vi "Add_Remove Point from Picture.vi"(6 "row index (0)":i32, 7 "2D Picture":refnum<vi>, 10 "draw options":T2={"Background Color"=16777215, "Grid Color"=13816530, "Angle Units"=enum."Degrees", "Draw Solid Background"=TRUE, "Draw Grid"=TRUE, "Grid Spacing"=0.25, "AutoScale"=FALSE, "Fit to Radius"=1.0, "data row options"=[]}, 11 "data in":T1) -> (0 "state changed?":bool, 1 "data changed?":bool, 3 "data out":T1)   [LabVIEW 2017, in "NI_Robotics_2D Rangefinder.xctl"]
uses:
  <vilib>/robotics/Controls/2D Rangefinder/NI_Robotics_2D Rangefinder.xctl
  <vilib>/robotics/Controls/2D Rangefinder/2D Rangefinder Picture/Draw Options.ctl
  <vilib>/robotics/Controls/Utilities/Angle Units.ctl
  <vilib>/robotics/Controls/2D Rangefinder/2D Rangefinder Picture/Data Row Options.ctl
  <vilib>/robotics/Controls/2D Rangefinder/2D Rangefinder Picture/Rangefinder Data.ctl
  <vilib>/robotics/Controls/2D Rangefinder/2D Rangefinder Picture/NI_Robotics_2D Rangefinder Picture.lvlib
  <vilib>/robotics/Controls/Utilities/NI_Robotics_Control Utilities.lvlib
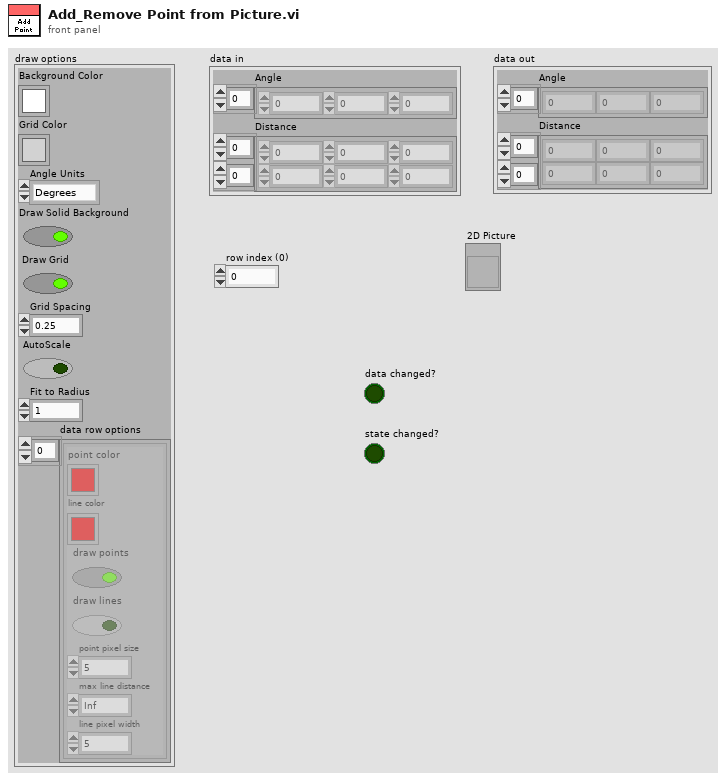
[diagram p1: front panel]
types:
  T1 = typedef "NI_Robotics_2D Rangefinder Picture.lvlib/Rangefinder Data.ctl" = cluster{"Angle":dbl[], "Distance":dbl[][]}
  T2 = typedef "NI_Robotics_2D Rangefinder Picture.lvlib/Draw Options.ctl" = cluster{"Background Color":u32, "Grid Color":u32, "Angle Units":T3, "Draw Solid Background":bool, "Draw Grid":bool, "Grid Spacing":dbl, "AutoScale":bool, "Fit to Radius":dbl, "data row options":T4[]}
  T3 = typedef "NI_Robotics_Control Utilities.lvlib/Angle Units.ctl" = enum16{"Radians", "Degrees"}
  T4 = typedef "NI_Robotics_2D Rangefinder Picture.lvlib/Data Row Options.ctl" = cluster{"point color":u32, "line color":u32, "draw points":bool, "draw lines":bool, "point pixel size":u16, "max line distance":dbl, "line pixel width":u16}
  T5 = typedef "LVBoundsTypeDef.ctl" = cluster{"Width":u32, "Height":u32}
  T6 = typedef "LVMouseTypeDef.ctl" = cluster{"Mouse Position":cluster{"X":i32, "Y":i32}, "Mouse Modifiers":cluster{"Button Down":bool, "Shift Mod":bool, "Menu Mod":bool, "Option Mod":bool}}
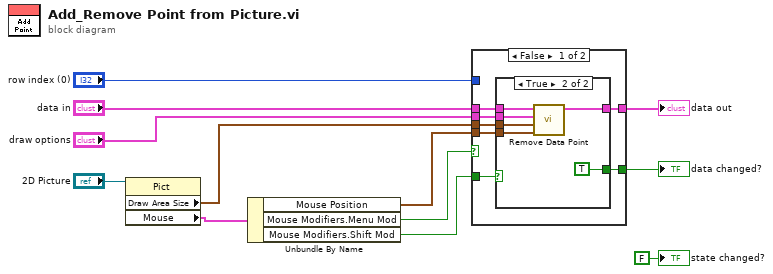
[diagram p0: block diagram]
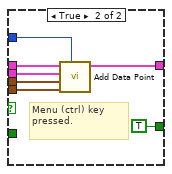
[diagram p3: hidden frame]
diagram:
  n1 = property class="Pict"(reference="2D Picture") -> ("Draw Area Size"=w10:T5, "Mouse"=w12:T6)  [unwired: 1 in, 2 out]
  n2 = Unbundle By Name(w12) -> ("Mouse Position"=w9:cluster{"X":i32, "Y":i32}, "Mouse Modifiers.Menu Mod"=w8:bool, "Mouse Modifiers.Shift Mod"=w7:bool)
  n3 = case shown="False" w8 {
    tunnel: "data in" -> [w18 w33]
    tunnel: [w17 w32] -> w2
    tunnel: "draw options" -> [w16 w31]
    tunnel: w10 -> [w15 w30]
    tunnel: w9 -> [w14 w29]
    tunnel: w7 -> [w19 _]
    tunnel: [w13 TRUE ("data changed?")] -> w5
    tunnel: "row index (0)" -> [_ w27]
    frame False {
      n4 = case shown="True" w19 {
        tunnel: w18 -> [w20 w25]
        tunnel: [w20 w24] -> w17
        tunnel: w16 -> [_ w23]
        tunnel: w15 -> [_ w22]
        tunnel: w14 -> [_ w21]
        tunnel: [_ TRUE ("data changed?")] -> w13
        frame False {
        }
        frame True {
          n5 = call <vilib>:"Remove Data Point.vi"("pixel position"=w21, "DrawAreaSize"=w22, "draw options"=w23, "data in"=w25) -> ("data out"=w24:T1)  [unwired: 7 in]
        }
      }
    }
    frame True {
      # "Menu (ctrl) key pressed."
      n6 = call <vilib>:"Add Data Point.vi"("row index (0)"=w27, "pixel position"=w29, "DrawAreaSize"=w30, "draw options"=w31, "data in"=w33) -> ("data out"=w32:T1)  [unwired: 6 in]
    }
  }
  "data changed?" <- w5
  "data out" <- w2
  "state changed?" <- FALSE ("state changed?")
